vi "Read Message Priority.vi"(8 "error in (no error)":errorcluster, 11 "Sequencer Msg in":refnum<class "Sequencer Msg.lvclass">) -> (0 "error out":errorcluster, 2 "Priority":u16=1, 3 "Sequencer Msg out":refnum<class "Sequencer Msg.lvclass">)   [LabVIEW 2020, in "Sequencer.lvlib" / "Sequencer Msg.lvclass"]
doc: "Read the Message Priority."
uses:
  Sequencer Msg.lvclass
  Sequencer Msg.lvclass/Sequencer Msg.ctl
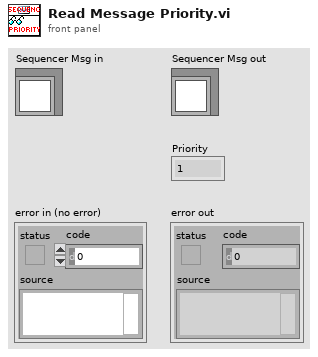
[diagram p1: front panel]
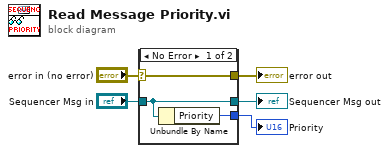
[diagram p0: block diagram]
diagram:
  n1 = case shown="No Error" "error in (no error)" {
    selector: "error in (no error)" -> [w8 w9]
    tunnel: [w8 w9] -> w4
    tunnel: [w7 w10] -> w2
    tunnel: "Sequencer Msg in" -> [w7 w10]
    tunnel: [w6 _] -> w1
    frame No Error {
      n2 = Unbundle By Name(w7) -> ("Priority"=w6:u16)
    }
    frame Error {
    }
  }
  "error out" <- w4
  "Sequencer Msg out" <- w2
  "Priority" <- w1
